vi "Create Calibration Results Summary Table.vi"(0 "Hysteresis Results":T4[](array[typedef]) {"Hysteresis Percent FS" format="%#_3g"}, 1 "Max Hysteresis %FS":dbl format="%#_3g", 2 "Accuracy Results":T3[](array[typedef]) {"Accuracy Percent FS" format="%#_3g"}, 3 "Max Accuracy %FS":dbl format="%#_3g", 4 "Repeatability Results":T2[](array[typedef]) {"Repeatability Percent FS" format="%#_3g"}, 5 "Max Repeatability %FS":dbl format="%#_3g", 6 "Linearity Results":T1[](array[typedef]) {"Linearity Percent FS" format="%#_3g"}, 7 "Max Linearity %FS":dbl format="%#_3g", 8 "Overall PassFail":bool, 9 "error in (no error)":errorcluster) -> (19 "error out":errorcluster, 20 "Session Table":string[][](array[string]))   [LabVIEW 2026, in "Analysis.lvlib"]
uses:
  Analysis.lvlib
  Hysteresis Result.ctl
  Accuracy Result.ctl
  Repeatability Result.ctl
  Linearity Result.ctl
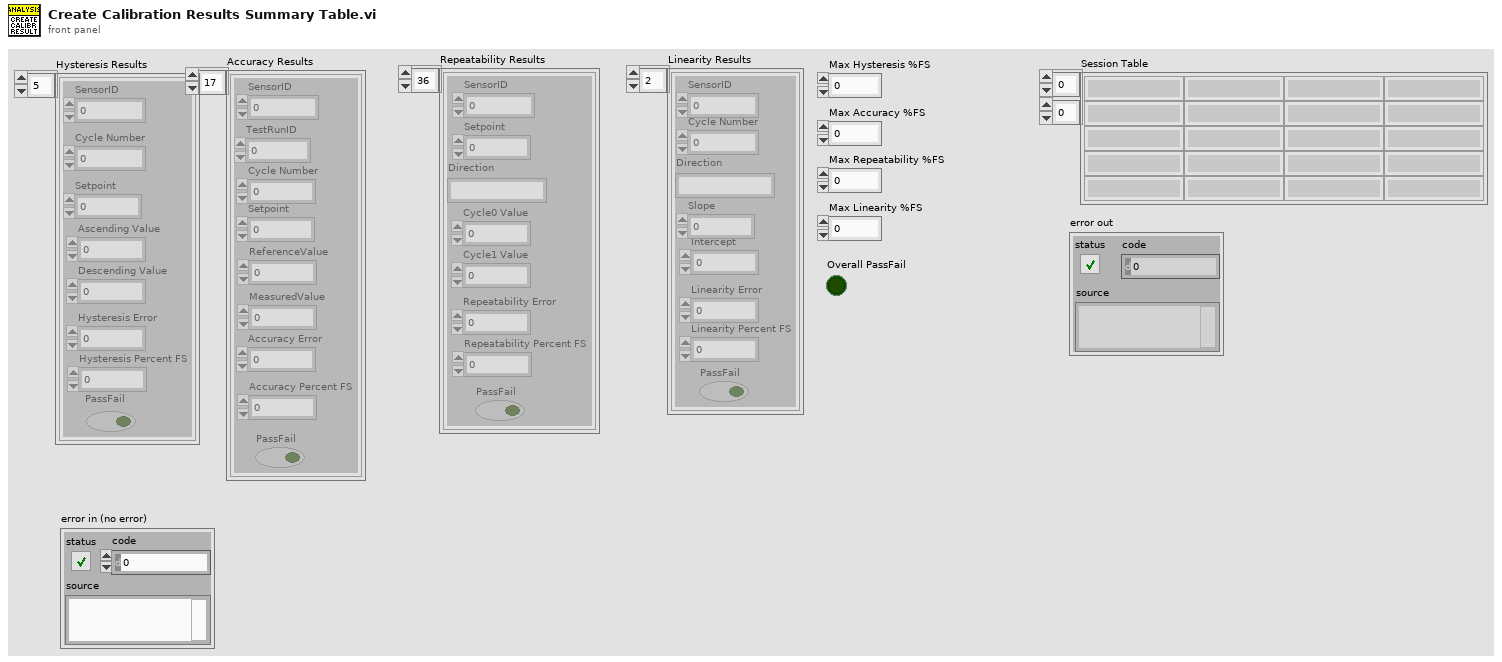
[diagram p1: front panel]
types:
  T1 = typedef "Analysis.lvlib/Linearity Result.ctl" = cluster{"Slope":dbl, "Intercept":dbl, "Cycle Number":i32, "SensorID":i32, "Linearity Error":dbl, "Linearity Percent FS":dbl, "Direction":string, "PassFail":bool}
  T2 = typedef "Analysis.lvlib/Repeatability Result.ctl" = cluster{"Setpoint":dbl, "Cycle0 Value":dbl, "SensorID":i32, "Cycle1 Value":dbl, "Repeatability Error":dbl, "Direction":string, "Repeatability Percent FS":dbl, "PassFail":bool}
  T3 = typedef "Analysis.lvlib/Accuracy Result.ctl" = cluster{"Setpoint":dbl, "Cycle Number":i32, "SensorID":i32, "TestRunID":i32, "ReferenceValue":dbl, "MeasuredValue":dbl, "Accuracy Percent FS":dbl, "PassFail":bool, "Accuracy Error":dbl}
  T4 = typedef "Analysis.lvlib/Hysteresis Result.ctl" = cluster{"Setpoint":dbl, "Ascending Value":dbl, "Cycle Number":i32, "SensorID":i32, "Descending Value":dbl, "Hysteresis Error":dbl, "Hysteresis Percent FS":dbl, "PassFail":bool}
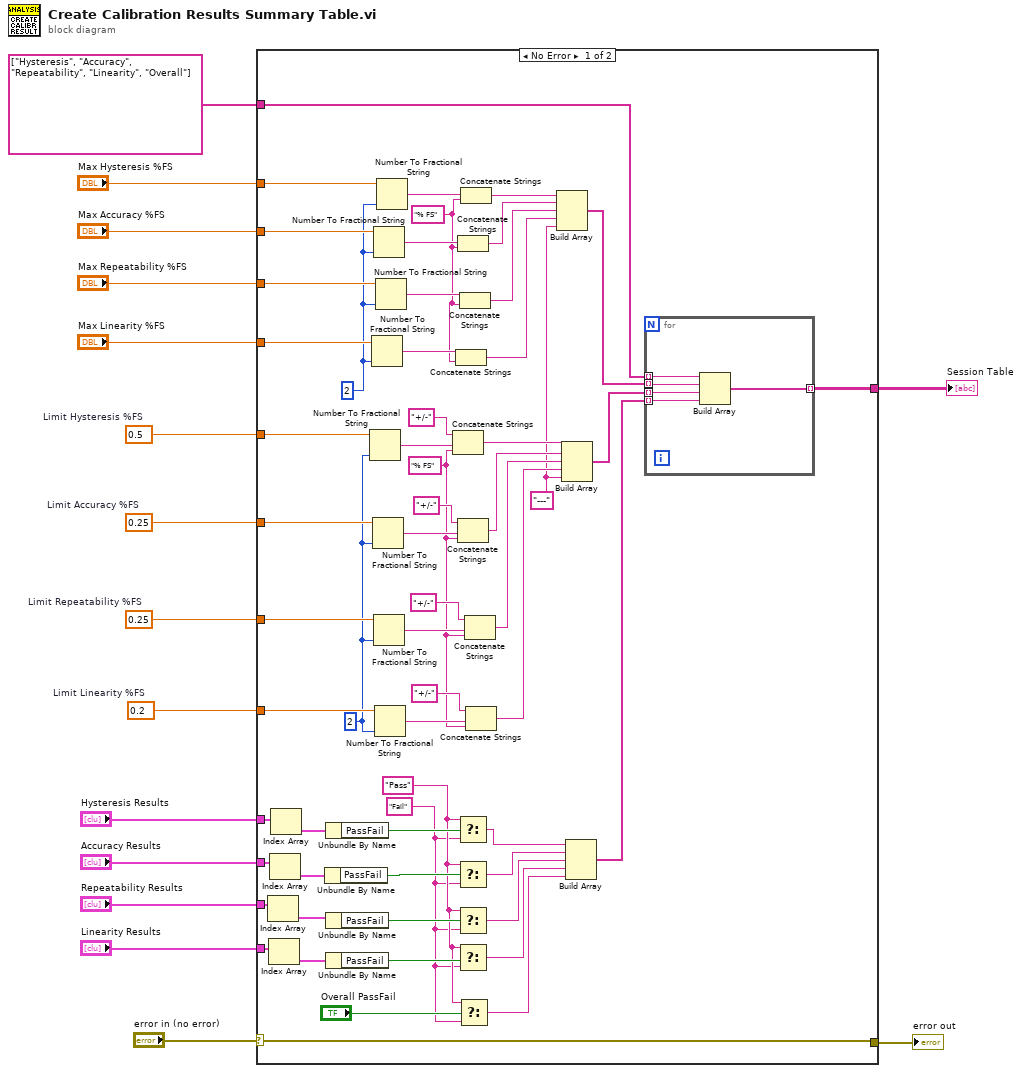
[diagram p0: block diagram]
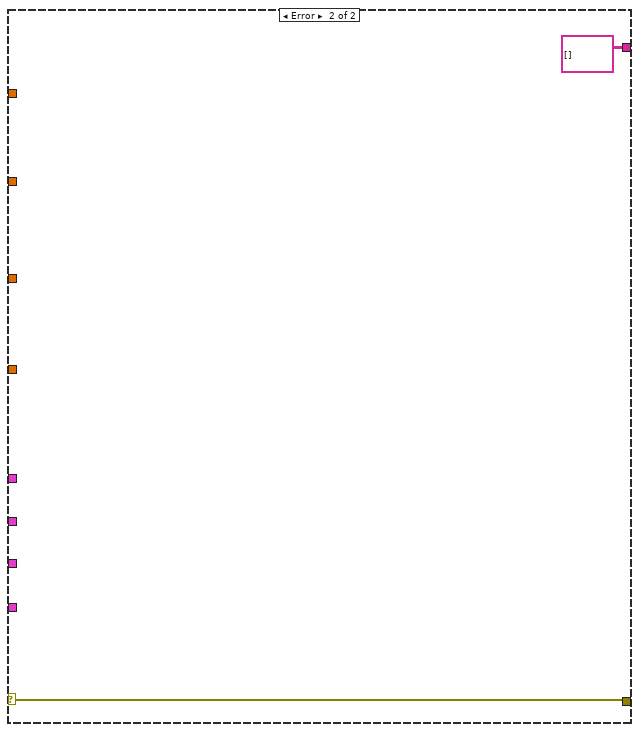
[diagram p2: hidden frame]
diagram:
  w9 = 0.2  # Limit Linearity %FS
  w10 = 0.25  # Limit Repeatability %FS
  w11 = 0.25  # Limit Accuracy %FS
  w12 = 0.5  # Limit Hysteresis %FS
  n1 = case shown="No Error" "error in (no error)" {
    selector: "error in (no error)" -> [w17 w81]
    tunnel: "Max Hysteresis %FS" -> [w75 _]
    tunnel: "Max Accuracy %FS" -> [w71 _]
    tunnel: "Max Repeatability %FS" -> [w69 _]
    tunnel: "Max Linearity %FS" -> [w65 _]
    tunnel: w12 -> [w63 _]
    tunnel: w11 -> [w57 _]
    tunnel: w10 -> [w53 _]
    tunnel: w9 -> [w49 _]
    tunnel: "Hysteresis Results" -> [w47 _]
    tunnel: "Accuracy Results" -> [w46 _]
    tunnel: "Repeatability Results" -> [w45 _]
    tunnel: "Linearity Results" -> [w44 _]
    tunnel: string[] ["Hysteresis", "Accuracy", "Repeatability", "Linearity", "Overall"] ("element") -> [w31 _]
    tunnel: [w22 string[][] []] -> w3
    tunnel: [w17 w81] -> w1
    frame No Error {
      w20 = i16 2 ("precision (6)")
      w21 = i16 2 ("width (-)")
      w23 = "---" ("element")
      w25 = "Fail" ("element")
      w26 = "Pass" ("element")
      w18 = "% FS" ("element")
      w19 = "% FS" ("element")
      n2 = Index Array(array=w45) -> (element=w41:T2)  [unwired: 1 in]
      n3 = Index Array(array=w44) -> (element=w40:T1)  [unwired: 1 in]
      n4 = Index Array(array=w46) -> (element=w42:T3)  [unwired: 1 in]
      n5 = Index Array(array=w47) -> (element=w43:T4)  [unwired: 1 in]
      n6 = Unbundle By Name(w42) -> ("PassFail"=w38:bool)
      n7 = Unbundle By Name(w43) -> ("PassFail"=w39:bool)
      n8 = Unbundle By Name(w41) -> ("PassFail"=w37:bool)
      n9 = Unbundle By Name(w40) -> ("PassFail"=w36:bool)
      n10 = Number To Fractional String(number=w63, precision (6)=w21) -> (F-format string=w62:string)  [unwired: 2 in]
      n11 = Number To Fractional String(number=w65, precision (6)=w20) -> (F-format string=w66:string)  [unwired: 2 in]
      n12 = Number To Fractional String(number=w57, precision (6)=w21) -> (F-format string=w59:string)  [unwired: 2 in]
      n13 = Number To Fractional String(number=w71, precision (6)=w20) -> (F-format string=w72:string)  [unwired: 2 in]
      n14 = Number To Fractional String(number=w53, precision (6)=w21) -> (F-format string=w55:string)  [unwired: 2 in]
      n15 = Number To Fractional String(number=w49, precision (6)=w21) -> (F-format string=w51:string)  [unwired: 2 in]
      n16 = Number To Fractional String(number=w69, precision (6)=w20) -> (F-format string=w68:string)  [unwired: 2 in]
      n17 = Number To Fractional String(number=w75, precision (6)=w20) -> (F-format string=w74:string)  [unwired: 2 in]
      n18 = Concatenate Strings("+/-" ("element"), w62, w18) -> (w61:string)
      n19 = Concatenate Strings(w66, w19) -> (w64:string)
      n20 = Concatenate Strings(w72, w19) -> (w70:string)
      n21 = Concatenate Strings("+/-" ("element"), w59, w18) -> (w56:string)
      n22 = Select(t=w26, s=w39, f=w25) -> (s? t:f=w35:string)
      n23 = Select(t=w26, s=w38, f=w25) -> (s? t:f=w34:string)
      n24 = Select(t=w26, s=w37, f=w25) -> (s? t:f=w33:string)
      n25 = Select(t=w26, s=w36, f=w25) -> (s? t:f=w32:string)
      n26 = Select(t=w26, s="Overall PassFail", f=w25) -> (s? t:f=w24:string)
      n27 = Concatenate Strings(w68, w19) -> (w67:string)
      n28 = Concatenate Strings(w74, w19) -> (w73:string)
      n29 = Concatenate Strings("+/-" ("element"), w55, w18) -> (w52:string)
      n30 = Concatenate Strings("+/-" ("element"), w51, w18) -> (w48:string)
      n31 = Build Array(w73, w70, w67, w64, w23) -> (w30:string[])
      n32 = Build Array(w61, w56, w52, w48, w23) -> (w29:string[])
      n33 = Build Array(w35, w34, w33, w32, w24) -> (w28:string[])
      n34 = for {
        tunnel: w31 -> [w80] mode=indexing
        tunnel: w30 -> [w79] mode=indexing
        tunnel: w29 -> [w78] mode=indexing
        tunnel: w28 -> [w77] mode=indexing
        tunnel: [w76] -> w22 mode=indexing
        n35 = Build Array(w80, w79, w78, w77) -> (w76:string[])
      }
    }
    frame Error {
    }
  }
  "Session Table" <- w3
  "error out" <- w1
